vi "Set VI Color.vi"(10 "Pane Color":u32, 11 "VI in":refnum<vi>) -> ()   [LabVIEW 2013, in "main.lvlib"]
uses:
  main.lvlib
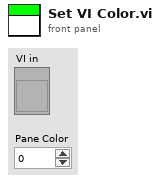
[diagram p1: front panel]
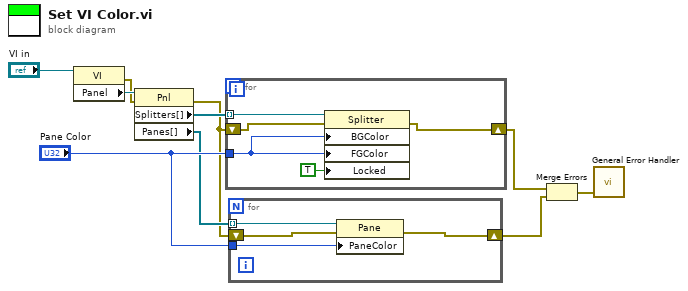
[diagram p0: block diagram]
diagram:
  n1 = property class="VI"(reference="VI in") -> (error out=w2:errorcluster, "Panel"=w8:refnum<vi>)  [unwired: 1 in, 1 out]
  n2 = property class="Pnl"(reference=w8, error in=w2) -> (error out=w1:errorcluster, "Splitters[]"=w9:refnum<vi>[], "Panes[]"=w6:refnum<vi>[])  [unwired: 1 out]
  n3 = for {
    tunnel: w9 -> [w15] mode=indexing
    tunnel: "Pane Color" -> [w14]
    shift-right: [w11] -> w5
    shift-left: w1 -> [w12]
    n4 = property class="Splitter"(reference=w15, error in=w12, "BGColor"=w14, "FGColor"=w14, "Locked"=TRUE ("Splitter Position Locked")) -> (error out=w11:errorcluster)  [unwired: 1 out]
  }
  n5 = for {
    shift-right: [w19] -> w4
    shift-left: w1 -> [w18]
    tunnel: "Pane Color" -> [w17]
    tunnel: w6 -> [w16] mode=indexing
    n6 = property class="Pane"(reference=w16, error in=w18, "PaneColor"=w17) -> (error out=w19:errorcluster)  [unwired: 1 out]
  }
  n7 = Merge Errors(w5, w4) -> (w3:errorcluster)
  n8 = call <vilib>:"General Error Handler.vi"("error in (no error)"=w3) -> ()  [unwired: 10 in, 5 out]
